vi "LJM logger apply formula to array.vi"(0 "Index":i32, 1 "Input Values":dbl[][](array[numeric]) format="%.2f", 2 "Variables Input":string[](array[string])=["v1", "v2", "v3", "v4"], 3 "formula":string, 4 "error in (no error)":errorcluster) -> (5 "Output Values":dbl[](array[numeric]) format="%.2f", 6 "error out":errorcluster)   [LabVIEW 2026]
doc: "Similar to the Formula Node function, but with variables that can be entered on the front panel."
uses:
  <vilib>/gmath/NI_Gmath.lvlib
panel:
  in  "Variables Output":string[](array[string])=["y"]
  # "Input = v\nOutput = y"
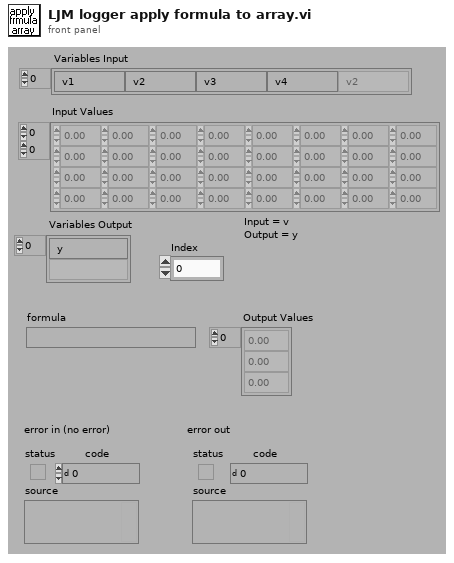
[diagram p1: front panel]
types:
  T1 = cluster{"Y Values":dbl[][], "Tables":i32[][][], "Variables input decode":i32[], "Variables output decode":i32[]}
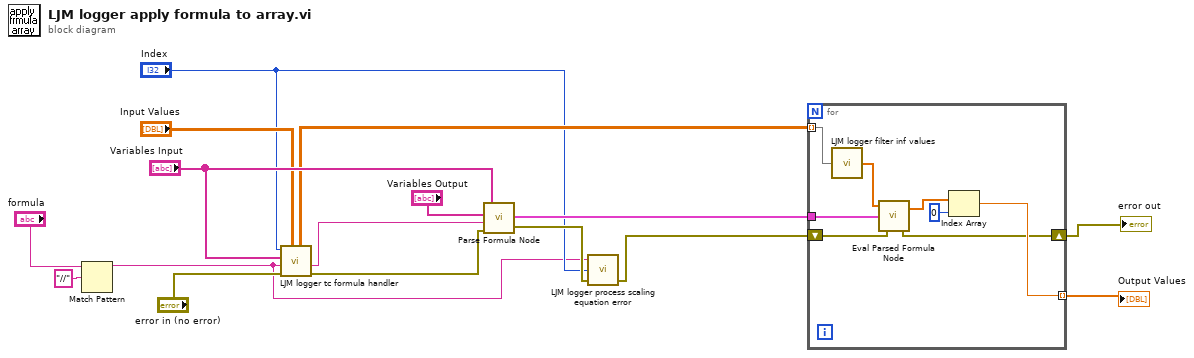
[diagram p0: block diagram]
diagram:
  n1 = Match Pattern(string="formula", regular expression="//") -> (before substring=w2:string)  [unwired: 1 in, 3 out]
  n2 = call "LJM logger tc formula handler.vi"("Input Values In"="Input Values", "error in (no error)"="error in (no error)", "formula"=w2, "Variables Input"="Variables Input", "Index"="Index") -> ("error out"=w6:errorcluster, "formula out"=w1:string, "Input Values Out"=w9:dbl[][])  [unwired: 2 in]
  n3 = call <vilib>:"Parse Formula Node.vi"("error in (no error)"=w6, "formula"=w1, "Variables Output"="Variables Output", "Variables Input"="Variables Input") -> ("error out"=w5:errorcluster, "Parsed Formula Node"=w15:T1)
  n4 = call "LJM logger process scaling equation error.vi"("Error In"=w5, "Scaling Equation Index"="Index", "Bad Formula"=w2) -> ("Error Out"=w4:errorcluster)  [unwired: 2 in]
  n5 = for {
    tunnel: w9 -> [w17] mode=indexing
    tunnel: w15 -> [w24]
    tunnel: [w21] -> w14 mode=indexing
    shift-right: [w19] -> w16
    shift-left: w4 -> [w20]
    n6 = call "LJM logger filter inf values.vi"("InValues"=w17) -> ("OutValues"=w18:dbl[])
    n7 = call <vilib>:"Eval Parsed Formula Node.vi"("error in (no error)"=w20, "Parsed Formula Node"=w24, "Input Values"=w18) -> ("error out"=w19:errorcluster, "Output Values"=w23:dbl[])
    n8 = Index Array(array=w23, index=0 ("Index")) -> (element=w21:dbl)
  }
  "Output Values" <- w14
  "error out" <- w16
